vi "create.vi"(8 "error in (no error)":errorcluster, 11 "Category Table":refnum<vi>) -> (0 "error out":errorcluster, 3 "CategoryListUIAdapter out":refnum<class "CategoryListUIAdapter.lvclass">)   [LabVIEW 2020, in "CategoryListUIAdapter.lvclass"]
uses:
  CategoryListUIAdapter.lvclass
  C:/GitRepos/Filthy-Lucre-Budgetizer/source/support/classes/AbstractMultiColumnListBoxAdapter/AbstractMultiColumnListBoxAdapter.lvclass
  CategoryListUIAdapter.lvclass/CategoryListUIAdapter.ctl
  AbstractMultiColumnListBoxAdapter/AbstractMultiColumnListBoxAdapter.lvclass
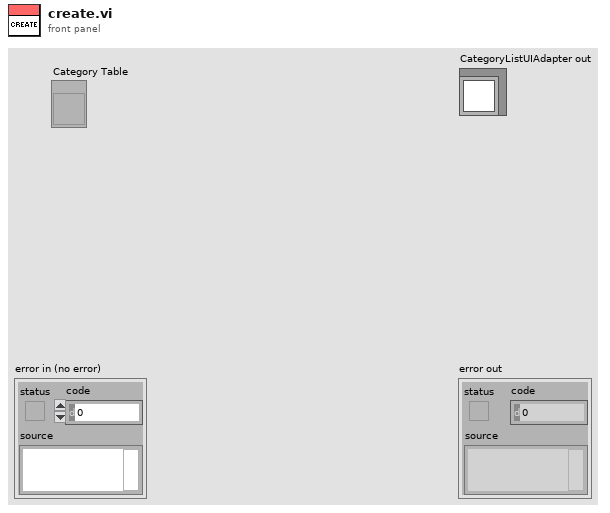
[diagram p1: front panel]
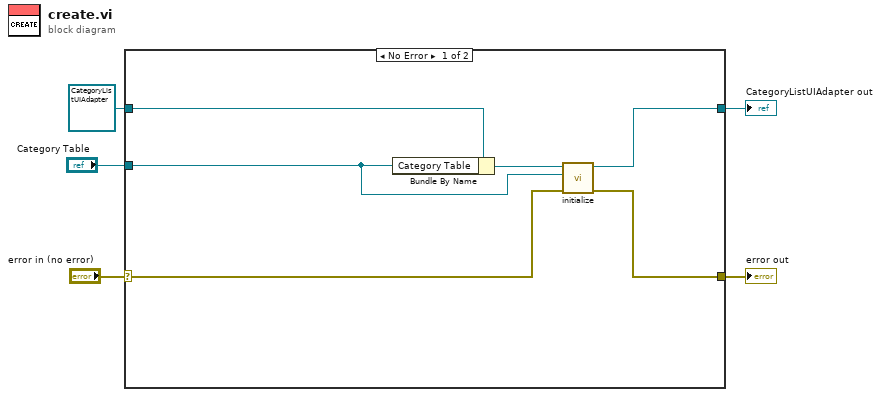
[diagram p0: block diagram]
diagram:
  n1 = case shown="No Error" "error in (no error)" {
    selector: "error in (no error)" -> [w7 w13]
    tunnel: [w6 w13] -> w4
    tunnel: [w9 w12] -> w3
    tunnel: refnum<class "CategoryListUIAdapter.lvclass"> refnum ("CategoryListUIAdapter in") -> [w11 w12]
    tunnel: "Category Table" -> [w8 _]
    frame No Error {
      n2 = Bundle By Name(cluster=w11, "Category Table"=w8) -> (w10:refnum<class "CategoryListUIAdapter.lvclass">)
      n3 = call "initialize.vi"("error in (no error)"=w7, "MCListbox Refnum"=w8, "AbstractMultiColumnListBoxAdapter in"=w10) -> ("error out"=w6:errorcluster, "AbstractMultiColumnListBoxAdapter out"=w9:refnum<class "CategoryListUIAdapter.lvclass">)  [unwired: 7 in]
    }
    frame Error {
    }
  }
  "error out" <- w4
  "CategoryListUIAdapter out" <- w3
